vi "日志报警状态存储 (子VI).vi"() -> ()   [LabVIEW 2016, in "斯坦道CODMn.lvlib"]
uses:
  <vilib>/ptbypt/NI_PtbyPt.lvlib
  <vilib>/Utility/config.llb/NI_LVConfig.lvlib
panel:
  out "多列列表框":i32(listbox)
  out "CODMn工作状态":T1(ring)
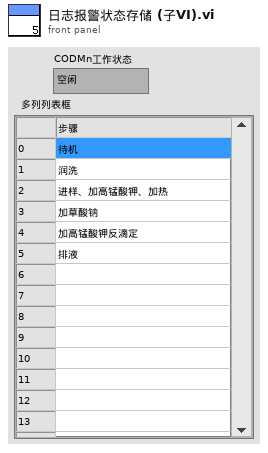
[diagram p1: front panel]
types:
  T1 = enum16{"空闲", "水样测试", "标样核查", "零点核查", "跨度核查", "空白测试", "平行样测试", "质控样", "空白校准", "标样校准", "加标回收"}
  T2 = cluster{"时间标识":timestamp, "设备":string, "日志信息":string}
  T3 = cluster{"时间标识":timestamp, "参数":string, "日志信息":string, "流程参数":string}
  T4 = cluster{"ORP故障":bool, "温控器故障":bool, "加热故障":bool, "高锰酸钾报警":bool, "草酸钠报警":bool, "测量错误":bool, "校零错误":bool, "校标错误":bool, " 进水样超量程":bool, "排液阀故障":bool}
  T5 = cluster{"时间标识":timestamp, "设备":string, "日志信息":string, "流程参数":string}
  T6 = cluster{"测量量程":dbl, "测量精度":dbl, "测量间隔":dbl, "消解温度":dbl, "消解时长":dbl, "空白校准时间":timestamp, "曲线截距":dbl, "曲线斜率":dbl, "测量检出限":dbl, "测量信号值":dbl, "线性相关系数":dbl, "二次多项式系数":dbl, "标样校准时间":timestamp, "单位":u16}
  T7 = typedef "NI_LVConfig.lvlib/Config Data RefNum.ctl" = refnum<k1>
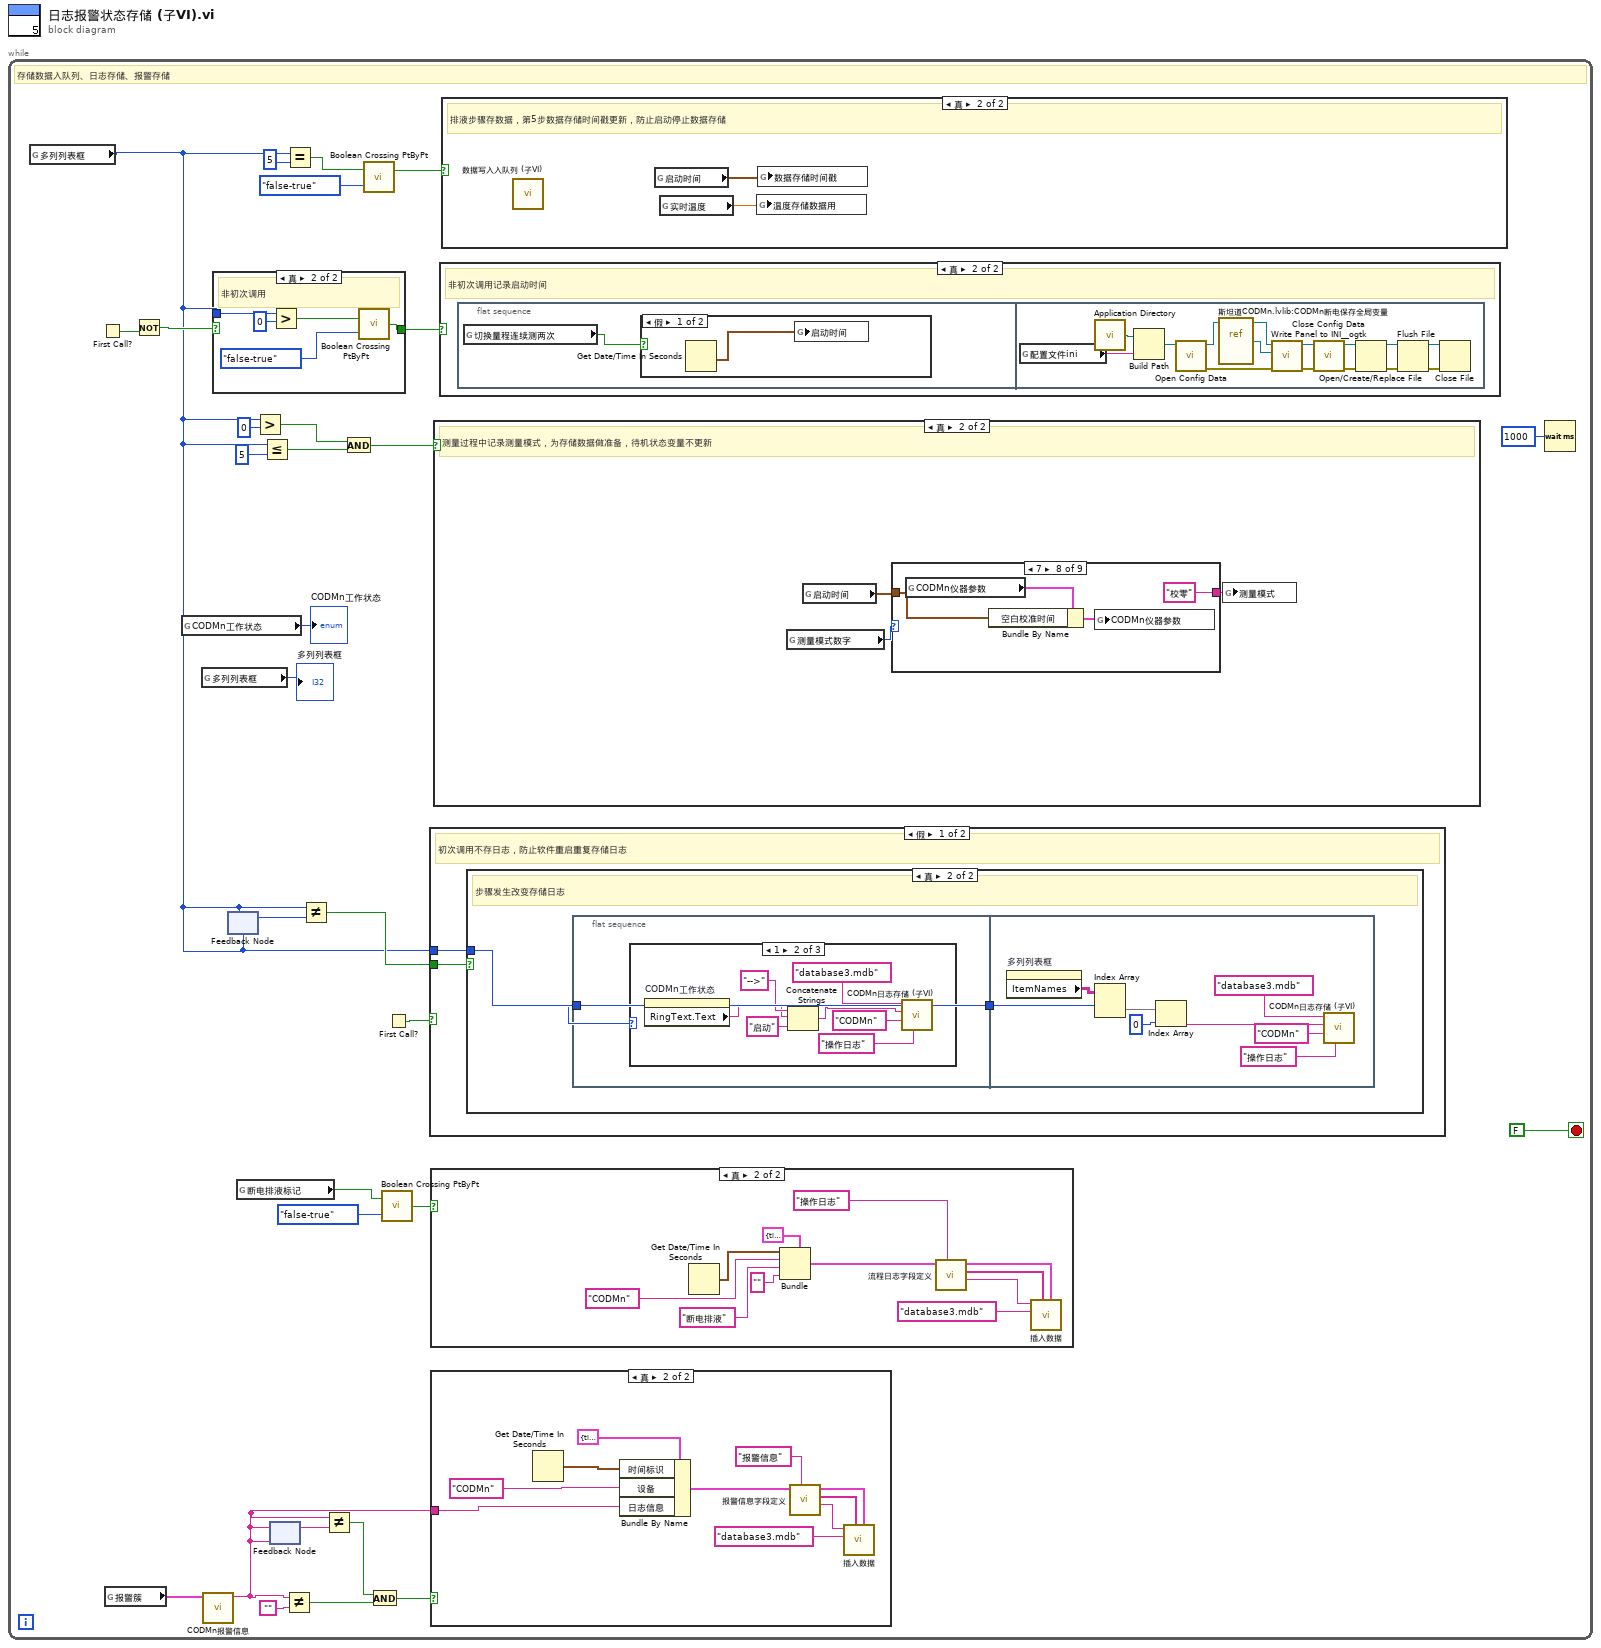
[diagram p0: block diagram]
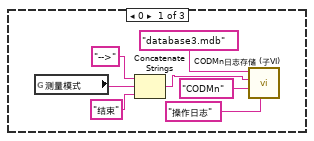
[diagram p3: hidden frame]
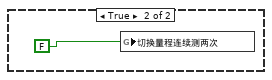
[diagram p10: hidden frame]
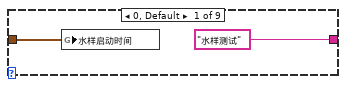
[diagram p12: hidden frame]
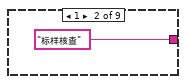
[diagram p13: hidden frame]
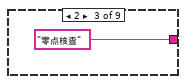
[diagram p14: hidden frame]
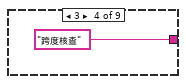
[diagram p15: hidden frame]
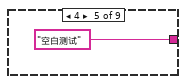
[diagram p16: hidden frame]
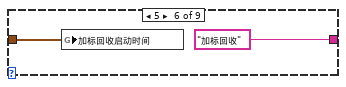
[diagram p17: hidden frame]
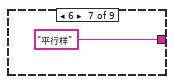
[diagram p18: hidden frame]
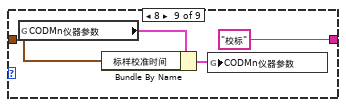
[diagram p19: hidden frame]
diagram:
  n1 = while {
    stop <- FALSE stop-if-true
    # "存储数据入队列、日志存储、报警存储"
    n2 = global read "运行时序全局变量.vi" "多列列表框"() -> (w5:i32)
    n3 = First Call?() -> (First Call?: T/F=w8:bool)
    n4 = global read "COD内部交互全局.vi" "报警簇"() -> (w4:T4)
    n5 = Not(x=w8) -> (.not. x?=w6:bool)
    n6 = global read "COD测量模式全局.vi" "CODMn工作状态"() -> (→"CODMn工作状态":T1)
    n7 = global read "运行时序全局变量.vi" "多列列表框"() -> (→"多列列表框":i32)
    n8 = call "CODMn报警信息.vi"("报警簇"=w4) -> ("CODMN报警信息"=w9:string)  [unwired: 10 in]
    n9 = case shown="真" w6 {
      selector: w6 -> [w58 _]
      tunnel: w5 -> [_ w60]
      tunnel: [w58 w59] -> w7
      frame False {
      }
      frame True {
        # "非初次调用"
        n10 = Greater?(x=w60, y=u16 0) -> (0:w63:bool)
        n11 = call <vilib>:"Boolean Crossing PtByPt.vi"("direction"=enum16{"either", "false-true", "true-false"}."false-true", "input"=w63) -> ("crossing"=w59:bool)  [unwired: 1 in]
      }
    }
    n12 = feedback #1(w5) -> (w19:i32)
    n13 = feedback-in #1(w5) -> ()
    n14 = global read "COD内部交互全局.vi" "断电排液标记"() -> (w3:bool)
    n15 = Greater?(x=w5, y=u16 0) -> (0:w30:bool)
    n16 = Less Or Equal?(x=w5, y=u16 5) -> (x <= y?=w27:bool)
    n17 = feedback #2(w9) -> (w10:string)
    n18 = feedback-in #2(w9) -> ()
    n19 = Not Equal?(x=w9, y="") -> (x != y?=w14:bool)
    n20 = Equal?(x=w5, y=u16 5) -> (x = y?=w23:bool)
    n21 = Not Equal?(x=w5, y=w19) -> (x != y?=w20:bool)
    n22 = Not Equal?(x=w9, y=w10) -> (x != y?=w11:bool)
    n23 = And(x=w30, y=w27) -> (x .and. y?=w28:bool)
    n24 = call <vilib>:"Boolean Crossing PtByPt.vi"("direction"=enum16{"either", "false-true", "true-false"}."false-true", "input"=w23) -> ("crossing"=w25:bool)  [unwired: 1 in]
    n25 = And(x=w11, y=w14) -> (x .and. y?=w12:bool)
    n26 = call <vilib>:"Boolean Crossing PtByPt.vi"("direction"=enum16{"either", "false-true", "true-false"}."false-true", "input"=w3) -> ("crossing"=w15:bool)  [unwired: 1 in]
    n27 = First Call?() -> (First Call?: T/F=w21:bool)
    n28 = case shown="假" w21 {
      tunnel: w20 -> [w32 _]
      tunnel: w5 -> [w31 _]
      frame False {
        # "初次调用不存日志，防止软件重启重复存储日志"
        n29 = case shown="真" w32 {
          tunnel: w31 -> [_ w34]
          frame False {
          }
          frame True {
            # "步骤发生改变存储日志"
            n30 = flat-sequence {
              tunnel: w34 -> [w35]
              tunnel: [w35] -> w33
              tunnel: w33 -> [w55]
              frame #0 {
                n31 = case shown="1" w35 {
                  frame 0 {
                    n32 = global read "COD测量模式全局.vi" "测量模式"() -> (w42:string)
                    n33 = Concatenate Strings("-->", w42, "结束" ("字符串")) -> (w41:string)
                    n34 = call "CODMn日志存储 (子VI).vi"("table输入"="操作日志", "参数"="CODMn" ("table输入"), "日志信息"=w41, "database"="database3.mdb") -> ()  [unwired: 8 in]
                  }
                  frame 1 {
                    n35 = property on="CODMn工作状态" class="Enum (严格)"() -> ("RingText.Text"=w43:string)  [unwired: 2 in, 2 out]
                    n36 = Concatenate Strings("-->", w43, "启动" ("字符串")) -> (w44:string)
                    n37 = call "CODMn日志存储 (子VI).vi"("table输入"="操作日志", "参数"="CODMn" ("table输入"), "日志信息"=w44, "database"="database3.mdb") -> ()  [unwired: 8 in]
                  }
                  frame 2, Default {
                  }
                }
              }
              frame #1 {
                n38 = property on="多列列表框" class="MCListbox (严格)"() -> ("ItemNames"=w50:string[][])  [unwired: 2 in, 2 out]
                n39 = Index Array(array=w50, index (row)=w55) -> (element=w53:string[])  [unwired: 1 in]
                n40 = Index Array(array=w53, index=0 ("索引")) -> (element=w51:string)
                n41 = call "CODMn日志存储 (子VI).vi"("table输入"="操作日志", "参数"="CODMn" ("table输入"), "日志信息"=w51, "database"="database3.mdb") -> ()  [unwired: 8 in]
              }
            }
          }
        }
      }
      frame True {
      }
    }
    n42 = case shown="真" w15 {
      frame False {
      }
      frame True {
        n43 = Get Date/Time In Seconds() -> (seconds since 1Jan1904=w79:timestamp)
        n44 = Bundle(cluster=T3 {"时间标识"=timestamp(0 s since 1904-01-01), "参数"="", "日志信息"="", "流程参数"=""} ("data in"), "时间标识"=w79, "参数"="CODMn" ("table输入"), "日志信息"="断电排液", "流程参数"="" ("table输入")) -> (w77:T3)
        n45 = call "流程日志字段定义.vi"("table输入"="操作日志", "data in"=w77) -> ("table输出"=w82:string, "columns"=w83:string[], "data out"=w84:T5)  [unwired: 7 in]
        n46 = call "插入数据.vi"("data"=w84, "columns"=w83, "database"="database3.mdb", "table"=w82) -> ()  [unwired: 7 in, 1 out]
      }
    }
    n47 = case shown="真" w12 {
      tunnel: w9 -> [_ w64]
      frame False {
      }
      frame True {
        n48 = Get Date/Time In Seconds() -> (seconds since 1Jan1904=w66:timestamp)
        n49 = Bundle By Name(cluster=T2 {"时间标识"=timestamp(0 s since 1904-01-01), "设备"="", "日志信息"=""} ("data in"), "时间标识"=w66, "设备"="CODMn", "日志信息"=w64) -> (w67:T2)
        n50 = call "报警信息字段定义.vi"("table输入"="报警信息", "data in"=w67) -> ("table输出"=w71:string, "columns"=w72:string[], "data out"=w73:T2)  [unwired: 7 in]
        n51 = call "插入数据.vi"("data"=w73, "columns"=w72, "database"="database3.mdb", "table"=w71) -> ()  [unwired: 7 in, 1 out]
      }
    }
    n52 = case shown="真" w28 {
      frame False {
      }
      frame True {
        # "测量过程中记录测量模式，为存储数据做准备，待机状态变量不更新"
        n53 = global read "COD内部交互全局.vi" "测量模式数字"() -> (w103:i32)
        n54 = global read "CODMn断电保存全局变量.vi" "启动时间"() -> (w102:timestamp)
        n55 = case shown="7" w103 {
          tunnel: ["水样测试" ("测量模式") "标样核查" ("测量模式") "零点核查" ("测量模式") "跨度核查" ("测量模式") "空白测试" ("测量模式") "加标回收" ("测量模式") "平行样" ("测量模式") "校零" ("测量模式") "校标" ("测量模式")] -> w104
          tunnel: w102 -> [w105 _ _ _ _ w111 _ w114 w118]
          frame 0, Default {
            n56 = global write "COD测量模式全局.vi" "水样启动时间"(w105) -> ()
          }
          frame 1 {
          }
          frame 2 {
          }
          frame 3 {
          }
          frame 4 {
          }
          frame 5 {
            n57 = global write "COD测量模式全局.vi" "加标回收启动时间"(w111) -> ()
          }
          frame 6 {
          }
          frame 7 {
            n58 = global read "CODMn断电保存全局变量.vi" "CODMn仪器参数"() -> (w116:T6)
            n59 = Bundle By Name(cluster=w116, "空白校准时间"=w114) -> (w115:T6)
            n60 = global write "CODMn断电保存全局变量.vi" "CODMn仪器参数"(w115) -> ()
          }
          frame 8 {
            n61 = global read "CODMn断电保存全局变量.vi" "CODMn仪器参数"() -> (w120:T6)
            n62 = Bundle By Name(cluster=w120, "标样校准时间"=w118) -> (w119:T6)
            n63 = global write "CODMn断电保存全局变量.vi" "CODMn仪器参数"(w119) -> ()
          }
        }
        n64 = global write "COD测量模式全局.vi" "测量模式"(w104) -> ()
      }
    }
    n65 = case shown="真" w7 {
      frame False {
      }
      frame True {
        # "非初次调用记录启动时间"
        n66 = flat-sequence {
          frame #0 {
            n67 = global read "COD内部交互全局.vi" "切换量程连续测两次"() -> (w85:bool)
            n68 = case shown="假" w85 {
              frame False {
                n69 = Get Date/Time In Seconds() -> (seconds since 1Jan1904=w86:timestamp)
                n70 = global write "CODMn断电保存全局变量.vi" "启动时间"(w86) -> ()
              }
              frame True {
                n71 = global write "COD内部交互全局.vi" "切换量程连续测两次"(FALSE ("切换量程连续测两次")) -> ()
              }
            }
          }
          frame #1 {
            n72 = global read "COD内部交互全局.vi" "配置文件ini"() -> (w88:string)
            n73 = call <vilib>:"Application Directory.vi"() -> ("Application Directory"=w101:path)
            n74 = Build Path(base path=w101, name or relative path=w88) -> (appended path=w100:path)
            n75 = call <vilib>:"Open Config Data.vi"("configuration file path"=w100) -> ("error out"=w96:errorcluster, "refnum"=w99:T7)  [unwired: 8 in, 1 out]
            n76 = vi-ref "斯坦道CODMn.lvlib:CODMn断电保存全局变量.vi"() -> (w98:refnum<vi>)
            n77 = call <userlib>:"Write Panel to INI__ogtk.vi"("error in (no error)"=w96, "VI ref"=w98, "refnum"=w99) -> ("error out"=w95:errorcluster, "refnum out"=w97:T7)  [unwired: 7 in]
            n78 = call <vilib>:"Close Config Data.vi"("error in (no error)"=w95, "refnum"=w97) -> ("error out"=w90:errorcluster, "file path"=w89:path)  [unwired: 8 in]
            n79 = Open/Create/Replace File(file path (use dialog)=w89, error in=w90) -> (refnum out=w93:refnum<file>, error out=w94:errorcluster)  [unwired: 4 in, 1 out]
            n80 = Flush File(refnum=w93, error in=w94) -> (refnum out=w92:refnum<file>, error out=w91:errorcluster)
            n81 = Close File(refnum=w92, error in=w91) -> ()  [unwired: 2 out]
          }
        }
      }
    }
    n82 = case shown="真" w25 {
      frame False {
      }
      frame True {
        # "排液步骤存数据，第5步数据存储时间戳更新，防止启动停止数据存储"
        n83 = call "数据写入入队列 (子VI).vi"() -> ()  [unwired: 12 in]
        n84 = global read "CODMn断电保存全局变量.vi" "启动时间"() -> (w123:timestamp)
        n85 = global read "COD内部交互全局.vi" "实时温度"() -> (w122:dbl)
        n86 = global write "COD内部交互全局.vi" "温度存储数据用"(w122) -> ()
        n87 = global write "COD内部交互全局.vi" "数据存储时间戳"(w123) -> ()
      }
    }
    n88 = Wait (ms)(milliseconds to wait=u32 1000 ("等待时间（毫秒）")) -> ()  [unwired: 1 out]
  }
